vi "UpdateMotors.vi"(0 "I/O":T24 {"IMU SPI A"."SPI Configuration"."Frame Length" min=1 max=16}, 2 "Speed Fraction":dbl min=-1.0 max=1.0 step=0.01, 3 "Spin Fraction":dbl min=-1.0 max=1.0 step=0.001) -> ()   [LabVIEW 2015]
uses:
  <vilib>/myRIO/Instrument Drivers/Onboard IO/PWM/typedefs/PWM Reference.ctl
  <vilib>/myRIO/Common/Instrument Driver Framework/Utilities/typedefs/myRIO Generic Hardware Reference.ctl
  <vilib>/myRIO/Common/Instrument Driver Framework/Utilities/typedefs/Hardware Version Enum.ctl
  <vilib>/myRIO/Common/Instrument Driver Framework/Utilities/typedefs/myRIO v1.0 Reference.ctl
  <vilib>/myRIO/Common/Instrument Driver Framework/Utilities/typedefs/Generic FPGA Reference.ctl
  <vilib>/myRIO/Common/Instrument Driver Framework/myRIO v1.0/PWM/typedefs/PWM Channels Enum.ctl
  <vilib>/myRIO/Instrument Drivers/Onboard IO/PWM/typedefs/PWM Configuration.ctl
  <vilib>/myRIO/Instrument Drivers/Onboard IO/Encoder/typedefs/Encoder Reference.ctl
  <vilib>/myRIO/Common/Instrument Driver Framework/myRIO v1.0/Encoder/typedefs/Encoder Channels Enum.ctl
  <vilib>/myRIO/Instrument Drivers/Onboard IO/SPI/typedefs/SPI Reference.ctl
  <vilib>/myRIO/Common/Instrument Driver Framework/myRIO v1.0/SPI/typedefs/SPI Channels Enum.ctl
  <vilib>/myRIO/Instrument Drivers/Onboard IO/SPI/typedefs/SPI Configuration.ctl
  <vilib>/myRIO/Common/Instrument Driver Framework/myRIO v1.0/SPI/typedefs/SPI Clock Phase.ctl
  <vilib>/myRIO/Common/Instrument Driver Framework/myRIO v1.0/SPI/typedefs/SPI Clock Polarity.ctl
  <vilib>/myRIO/Common/Instrument Driver Framework/myRIO v1.0/SPI/typedefs/SPI Data Direction.ctl
  <vilib>/myRIO/Common/Instrument Driver Framework/myRIO v1.0/SPI/typedefs/SPI Frame Length.ctl
  <vilib>/myRIO/Instrument Drivers/Onboard IO/DIO/typedefs/DIO Reference.ctl
  <vilib>/myRIO/Common/Instrument Driver Framework/myRIO v1.0/DIO/typedefs/DIO Channels List.ctl
  <vilib>/myRIO/Common/Instrument Driver Framework/myRIO v1.0/DIO/typedefs/DIO Channels Enum.ctl
  <vilib>/myRIO/Instrument Drivers/Onboard IO/I2C/typedefs/I2C Reference.ctl
  <vilib>/myRIO/Common/Instrument Driver Framework/myRIO v1.0/I2C/typedefs/I2C Channels Enum.ctl
  <vilib>/myRIO/Instrument Drivers/Onboard IO/I2C/typedefs/I2C Configuration.ctl
  <vilib>/myRIO/Instrument Drivers/Onboard IO/I2C/typedefs/I2C Transfer Rate.ctl
  <vilib>/myRIO/Instrument Drivers/Onboard IO/PWM/vis/Set Duty Cycle and Frequency.vi
  <vilib>/Utility/error.llb/Error Cluster From Error Code.vi
  <vilib>/myRIO/Common/Instrument Driver Framework/myRIO v1.0/PWM/vis/myRIO v1.0 Write PWM.vi
  <vilib>/myRIO/Instrument Drivers/Onboard IO/PWM/PWM.lvlib
  <vilib>/myRIO/Instrument Drivers/Onboard IO/I2C/I2C.lvlib
  <vilib>/myRIO/Instrument Drivers/Onboard IO/DIO/DIO.lvlib
  <vilib>/myRIO/Instrument Drivers/Onboard IO/SPI/SPI.lvlib
  <vilib>/myRIO/Instrument Drivers/Onboard IO/Encoder/Encoder.lvlib
panel:
  out "Array of RMotF and LMotF":dbl[][](array[numeric]) format="%#_2g"
  out "R Mot F":dbl(graph)
  out "L Mot F":dbl(graph)
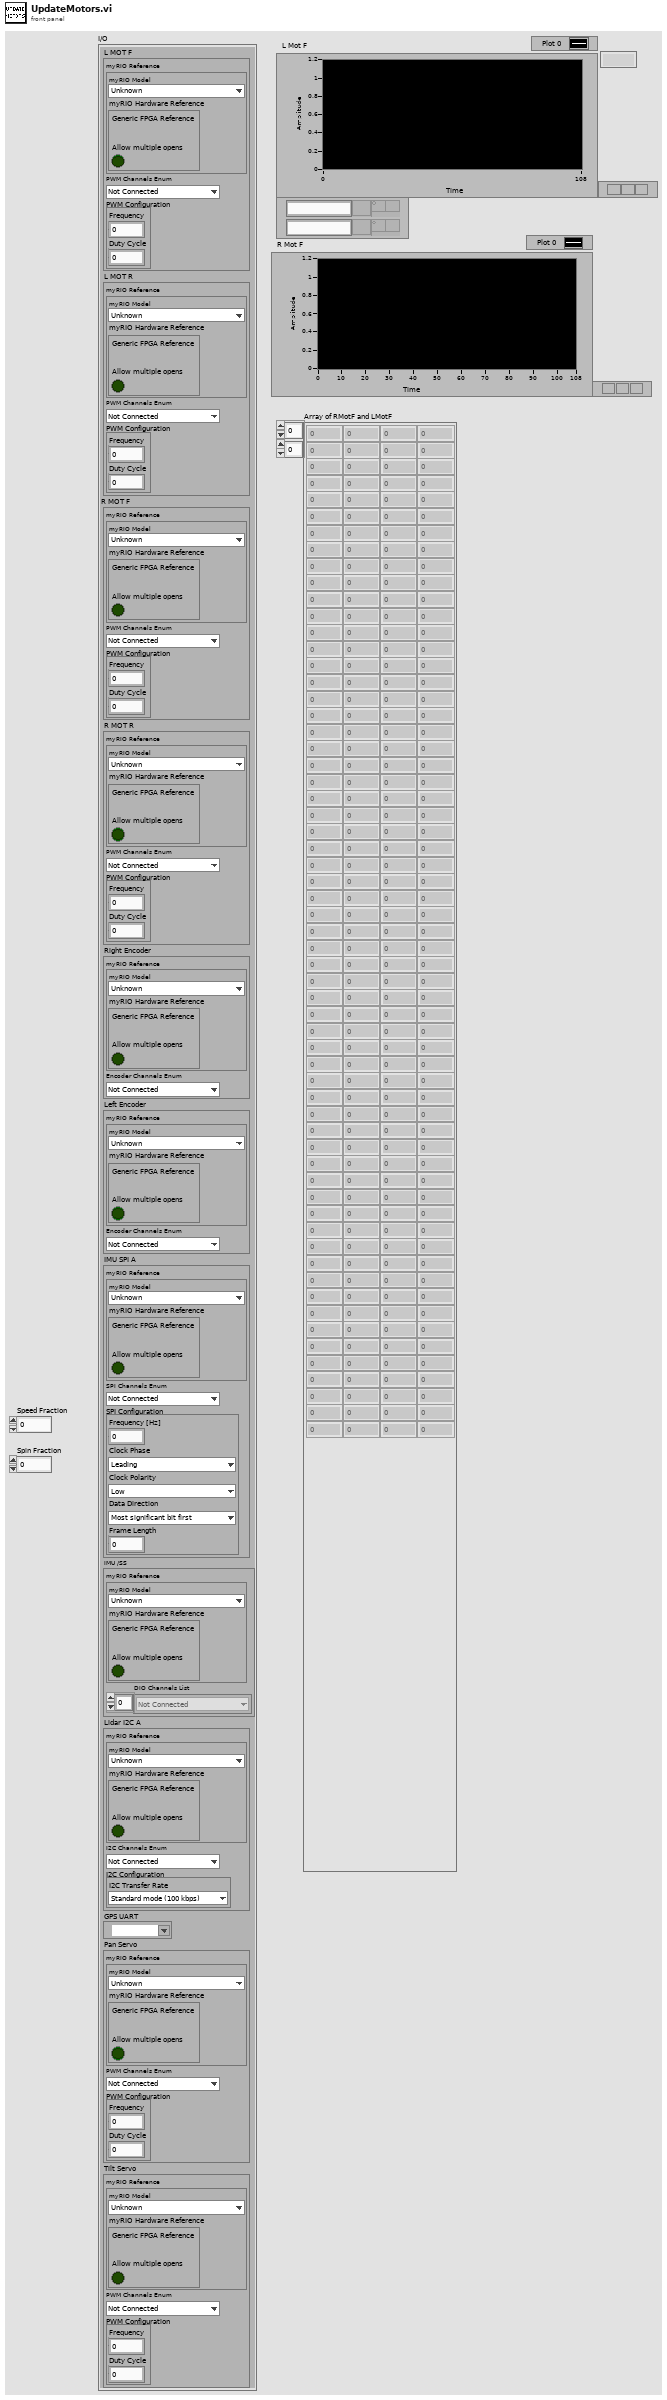
[diagram p1: front panel]
types:
  T1 = typedef "PWM.lvlib/PWM Reference.ctl" = cluster{"myRIO Reference":T2, "PWM Channels Enum":T6, "PWM Configuration":T7}
  T2 = typedef "myRIO Generic Hardware Reference.ctl" = cluster{"myRIO Model":T3, "myRIO Hardware Reference":T4}
  T3 = typedef "Hardware Version Enum.ctl" = enum16{"Unknown", "myRIO-1900", "myRIO-1950", "roboRIO"}
  T4 = typedef "myRIO v1.0 Reference.ctl" = cluster{"Generic FPGA Reference":T5, "Allow multiple opens":bool}
  T5 = typedef "Generic FPGA Reference.ctl" = refnum<k20>
  T6 = typedef "PWM Channels Enum.ctl" = enum16{"Not Connected", "C/PWM0", "C/PWM1", "A/PWM0", "A/PWM1", "A/PWM2", "B/PWM0", "B/PWM1", "B/PWM2", "PWM/PWM0", "PWM/PWM1", "PWM/PWM2", "PWM/PWM3", "PWM/PWM4", "PWM/PWM5", "PWM/PWM6", "PWM/PWM7", "PWM/PWM8", "PWM/PWM9"}
  T7 = typedef "PWM.lvlib/PWM Configuration.ctl" = cluster{"Frequency":dbl, "Duty Cycle":dbl}
  T8 = typedef "Encoder.lvlib/Encoder Reference.ctl" = cluster{"myRIO Reference":T2, "Encoder Channels Enum":T9}
  T9 = typedef "Encoder Channels Enum.ctl" = enum16{"Not Connected", "C/ENC0", "C/ENC1", "A/ENC", "B/ENC", "DIO/ENC0", "DIO/ENC1", "DIO/ENC2", "DIO/ENC3", "DIO/ENC4"}
  T10 = typedef "SPI.lvlib/SPI Reference.ctl" = cluster{"myRIO Reference":T2, "SPI Channels Enum":T11, "SPI Configuration":T12}
  T11 = typedef "SPI Channels Enum.ctl" = enum16{"Not Connected", "A/SPI", "B/SPI", "SPI/SPI"}
  T12 = typedef "SPI.lvlib/SPI Configuration.ctl" = cluster{"Frequency [Hz]":dbl, "Clock Phase":T13, "Clock Polarity":T14, "Data Direction":T15, "Frame Length":T16}
  T13 = typedef "SPI Clock Phase.ctl" = enum8{"Leading", "Trailing"}
  T14 = typedef "SPI Clock Polarity.ctl" = enum8{"Low", "High"}
  T15 = typedef "SPI Data Direction.ctl" = enum8{"Most significant bit first", "Least significant bit first"}
  T16 = typedef "SPI Frame Length.ctl" = u8
  T17 = typedef "DIO.lvlib/DIO Reference.ctl" = cluster{"myRIO Reference":T2, "DIO Channels List":T18}
  T18 = typedef "DIO Channels List.ctl" = T19[]
  T19 = typedef "DIO Channels Enum.ctl" = enum16{"Not Connected", "C/DIO0", "C/DIO1", "C/DIO2", "C/DIO3", "C/DIO4", "C/DIO5", "C/DIO6", "C/DIO7", "A/DIO0", "A/DIO1", "A/DIO2", "A/DIO3", "A/DIO4", "A/DIO5", "A/DIO6", "A/DIO7", "A/DIO8", "A/DIO9", "A/DIO10", "A/DIO11", "A/DIO12", "A/DIO13", "A/DIO14", "A/DIO15", "B/DIO0", "B/DIO1", "B/DIO2", "B/DIO3", "B/DIO4", "B/DIO5", "B/DIO6", "B/DIO7", "B/DIO8", "B/DIO9", "B/DIO10", "B/DIO11", "B/DIO12", "B/DIO13", "B/DIO14", "B/DIO15", "LED0", "LED1", "LED2", "LED3", "Button0", "DIO/DIO0", "DIO/DIO1", "DIO/DIO2", "DIO/DIO3", "DIO/DIO4", "DIO/DIO5", "DIO/DIO6", "DIO/DIO7", "DIO/DIO8", "DIO/DIO9", "SPI/CS0", "SPI/CS1", "SPI/CS2", "SPI/CS3", "LED RADIO (Green)", "LED RADIO (Red)", "LED COMM (Green)", "LED COMM (Red)", "LED MODE (Green)", "LED MODE (Red)"}
  T20 = typedef "I2C.lvlib/I2C Reference.ctl" = cluster{"myRIO Reference":T2, "I2C Channels Enum":T21, "I2C Configuration":T22}
  T21 = typedef "I2C Channels Enum.ctl" = enum16{"Not Connected", "A/I2C", "B/I2C", "I2C/I2C"}
  T22 = typedef "I2C.lvlib/I2C Configuration.ctl" = cluster{"I2C Transfer Rate":T23}
  T23 = typedef "I2C.lvlib/I2C Transfer Rate.ctl" = enum16{"Standard mode (100 kbps)", "Fast mode (400 kbps)"}
  T24 = cluster{"L MOT F":T1, "L MOT R":T1, "R MOT F":T1, "R MOT R":T1, "Right Encoder":T8, "Left Encoder":T8, "IMU SPI A":T10, "IMU /SS":T17, "Lidar I2C A":T20, "GPS UART":refnum<visa-resource-name>, "Pan Servo":T1, "Tilt Servo":T1}
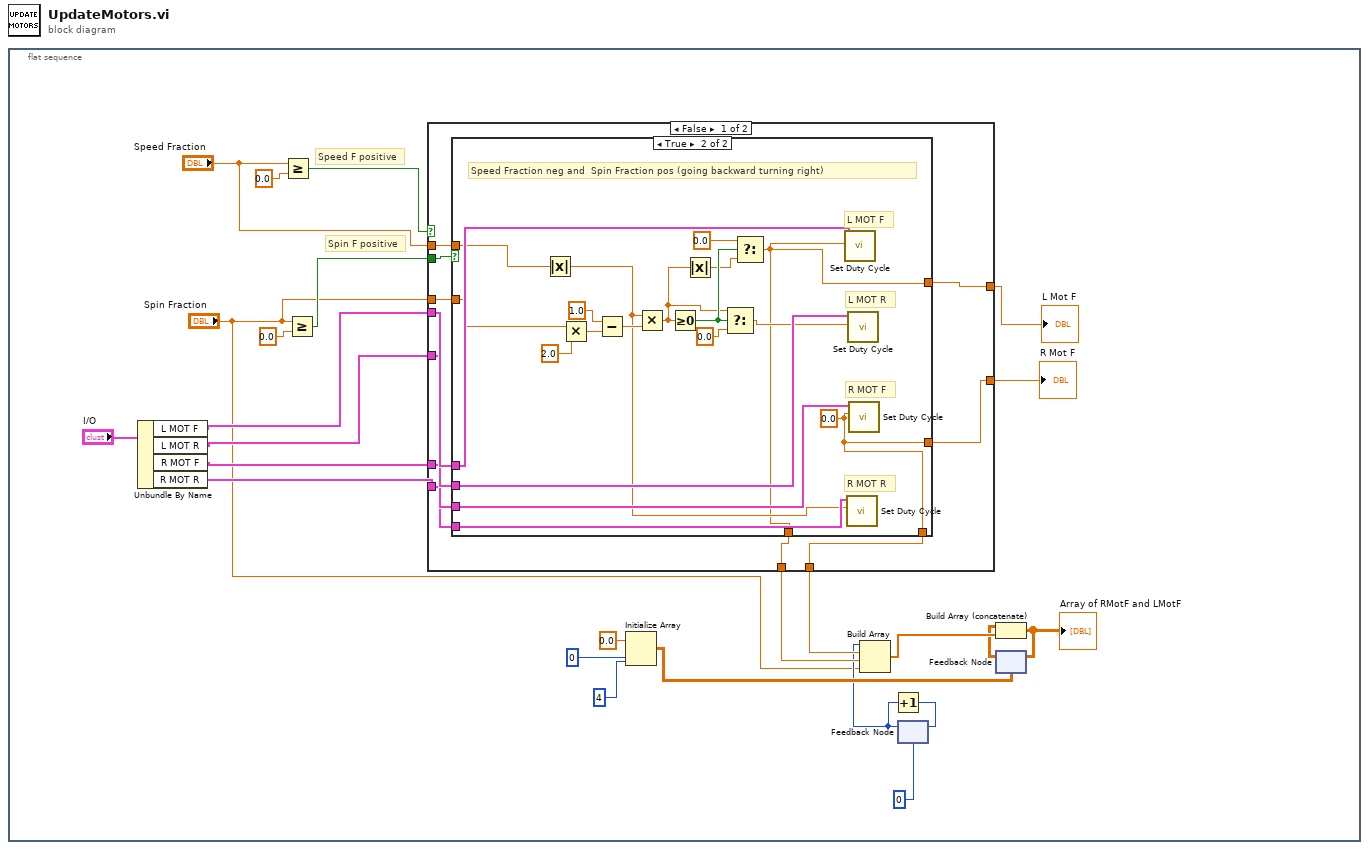
[diagram p0: block diagram]
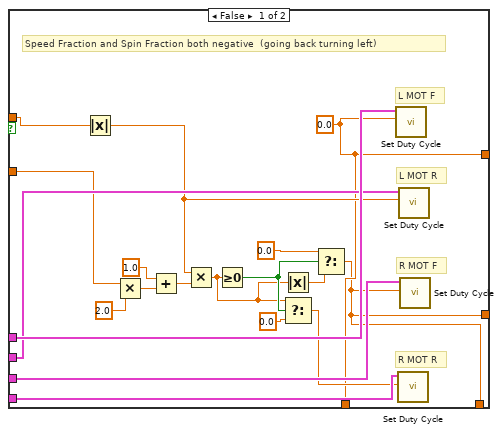
[diagram p2: hidden frame]
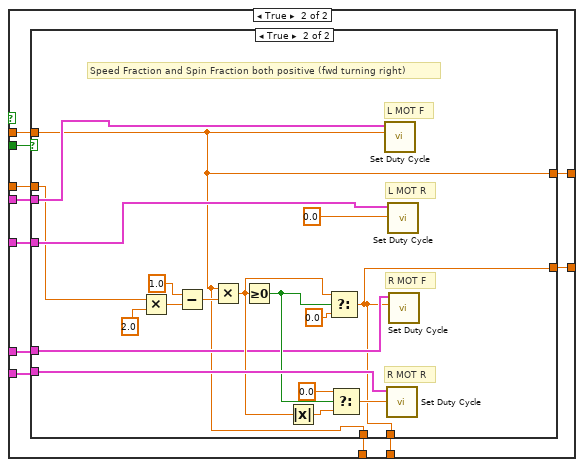
[diagram p3: hidden frame]
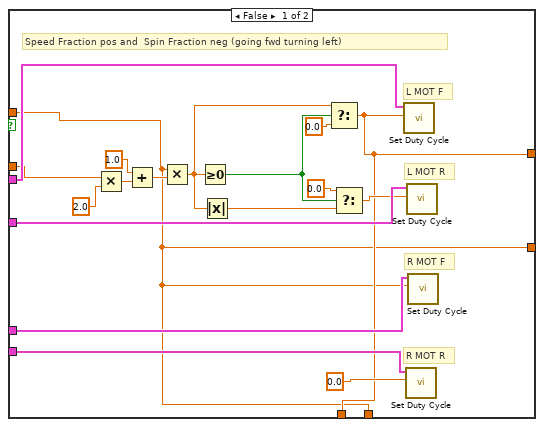
[diagram p4: hidden frame]
diagram:
  n1 = flat-sequence {
    frame #0 {
      # "Spin F positive"
      # "Speed F positive"
      n2 = Unbundle By Name("I/O") -> ("L MOT F"=w20:T1, "L MOT R"=w19:T1, "R MOT F"=w18:T1, "R MOT R"=w17:T1)
      n3 = Greater Or Equal?(x="Speed Fraction", y=0.0) -> (x >= y?=w23:bool)
      n4 = Greater Or Equal?(x="Spin Fraction", y=0.0) -> (x >= y?=w22:bool)
      n5 = case shown="False" w23 {
        tunnel: w22 -> [w36 w85]
        tunnel: w20 -> [w35 w84]
        tunnel: w19 -> [w34 w83]
        tunnel: w18 -> [w33 w82]
        tunnel: w17 -> [w32 w81]
        tunnel: [w31 w80] -> w16
        tunnel: [w30 w79] -> w15
        tunnel: [w28 w78] -> w13
        tunnel: [w29 w77] -> w12
        tunnel: "Speed Fraction" -> [w27 w76]
        tunnel: "Spin Fraction" -> [w26 w75]
        frame False {
          n6 = case shown="True" w36 {
            tunnel: w35 -> [w51 w70]
            tunnel: w34 -> [w50 w69]
            tunnel: w33 -> [w49 w68]
            tunnel: w32 -> [w48 w67]
            tunnel: [w40 w59] -> w31
            tunnel: [w39 w58] -> w30
            tunnel: [w40 w59] -> w29
            tunnel: [w39 w58] -> w28
            tunnel: w27 -> [w38 w57]
            tunnel: w26 -> [w37 w56]
            frame False {
              w40 = 0.0 ("Duty Cycle")
              # "Speed Fraction and Spin Fraction both negative  (going back turning left)"
              # "R MOT R"
              # "L MOT R"
              # "R MOT F"
              # "L MOT F"
              n7 = Absolute Value(x=w38) -> (abs(x)=w47:dbl)
              n8 = Multiply(x=w37, y=2.0) -> (x*y=w53:dbl)
              n9 = Add(x=1.0, y=w53) -> (x+y=w55:dbl)
              n10 = Multiply(x=w47, y=w55) -> (x*y=w42:dbl)
              n11 = Greater Or Equal To 0?(x=w42) -> (x >= 0?=w44:bool)
              n12 = Absolute Value(x=w42) -> (abs(x)=w41:dbl)
              n13 = Select(t=w42, s=w44, f=0.0) -> (s? t:f=w45:dbl)
              n14 = Select(t=0.0 ("Duty Cycle"), s=w44, f=w41) -> (s? t:f=w39:dbl)
              n15 = call <vilib>:"Set Duty Cycle.vi"("Duty Cycle"=w40, "PWM Ref In"=w51) -> ()  [unwired: 7 in, 2 out]
              n16 = call <vilib>:"Set Duty Cycle.vi"("Duty Cycle"=w45, "PWM Ref In"=w48) -> ()  [unwired: 7 in, 2 out]
              n17 = call <vilib>:"Set Duty Cycle.vi"("Duty Cycle"=w47, "PWM Ref In"=w50) -> ()  [unwired: 7 in, 2 out]
              n18 = call <vilib>:"Set Duty Cycle.vi"("Duty Cycle"=w39, "PWM Ref In"=w49) -> ()  [unwired: 7 in, 2 out]
            }
            frame True {
              w58 = 0.0 ("Duty Cycle")
              # "Speed Fraction neg and  Spin Fraction pos (going backward turning right)"
              # "R MOT R"
              # "L MOT R"
              # "R MOT F"
              # "L MOT F"
              n19 = Absolute Value(x=w57) -> (abs(x)=w66:dbl)
              n20 = Multiply(x=w56, y=2.0) -> (x*y=w73:dbl)
              n21 = Subtract(x=1.0, y=w73) -> (x-y=w71:dbl)
              n22 = Multiply(x=w66, y=w71) -> (x*y=w60:dbl)
              n23 = Greater Or Equal To 0?(x=w60) -> (x >= 0?=w62:bool)
              n24 = Absolute Value(x=w60) -> (abs(x)=w61:dbl)
              n25 = Select(t=w60, s=w62, f=0.0) -> (s? t:f=w65:dbl)
              n26 = Select(t=0.0 ("Duty Cycle"), s=w62, f=w61) -> (s? t:f=w59:dbl)
              n27 = call <vilib>:"Set Duty Cycle.vi"("Duty Cycle"=w59, "PWM Ref In"=w70) -> ()  [unwired: 7 in, 2 out]
              n28 = call <vilib>:"Set Duty Cycle.vi"("Duty Cycle"=w66, "PWM Ref In"=w67) -> ()  [unwired: 7 in, 2 out]
              n29 = call <vilib>:"Set Duty Cycle.vi"("Duty Cycle"=w65, "PWM Ref In"=w69) -> ()  [unwired: 7 in, 2 out]
              n30 = call <vilib>:"Set Duty Cycle.vi"("Duty Cycle"=w58, "PWM Ref In"=w68) -> ()  [unwired: 7 in, 2 out]
            }
          }
        }
        frame True {
          n31 = case shown="True" w85 {
            tunnel: w84 -> [w98 w116]
            tunnel: w83 -> [w97 w115]
            tunnel: w82 -> [w96 w107]
            tunnel: w81 -> [w95 w114]
            tunnel: [w88 w104] -> w80
            tunnel: [w87 w106] -> w79
            tunnel: [w87 w106] -> w78
            tunnel: [w88 w104] -> w77
            tunnel: w76 -> [w87 w104]
            tunnel: w75 -> [w86 w105]
            frame False {
              # "Speed Fraction pos and  Spin Fraction neg (going fwd turning left)"
              # "R MOT R"
              # "L MOT R"
              # "R MOT F"
              # "L MOT F"
              n32 = Multiply(x=w86, y=2.0) -> (x*y=w102:dbl)
              n33 = Add(x=1.0, y=w102) -> (x+y=w100:dbl)
              n34 = Multiply(x=w87, y=w100) -> (x*y=w90:dbl)
              n35 = Greater Or Equal To 0?(x=w90) -> (x >= 0?=w92:bool)
              n36 = Absolute Value(x=w90) -> (abs(x)=w89:dbl)
              n37 = Select(t=w90, s=w92, f=0.0) -> (s? t:f=w88:dbl)
              n38 = Select(t=0.0, s=w92, f=w89) -> (s? t:f=w93:dbl)
              n39 = call <vilib>:"Set Duty Cycle.vi"("Duty Cycle"=w88, "PWM Ref In"=w98) -> ()  [unwired: 7 in, 2 out]
              n40 = call <vilib>:"Set Duty Cycle.vi"("Duty Cycle"=0.0, "PWM Ref In"=w95) -> ()  [unwired: 7 in, 2 out]
              n41 = call <vilib>:"Set Duty Cycle.vi"("Duty Cycle"=w93, "PWM Ref In"=w97) -> ()  [unwired: 7 in, 2 out]
              n42 = call <vilib>:"Set Duty Cycle.vi"("Duty Cycle"=w87, "PWM Ref In"=w96) -> ()  [unwired: 7 in, 2 out]
            }
            frame True {
              # "Speed Fraction and Spin Fraction both positive (fwd turning right)"
              # "R MOT R"
              # "L MOT R"
              # "R MOT F"
              # "L MOT F"
              n43 = Multiply(x=w105, y=2.0) -> (x*y=w120:dbl)
              n44 = Subtract(x=1.0, y=w120) -> (x-y=w118:dbl)
              n45 = Multiply(x=w104, y=w118) -> (x*y=w109:dbl)
              n46 = Greater Or Equal To 0?(x=w109) -> (x >= 0?=w112:bool)
              n47 = Absolute Value(x=w109) -> (abs(x)=w110:dbl)
              n48 = Select(t=w109, s=w112, f=0.0) -> (s? t:f=w106:dbl)
              n49 = Select(t=0.0, s=w112, f=w110) -> (s? t:f=w108:dbl)
              n50 = call <vilib>:"Set Duty Cycle.vi"("Duty Cycle"=w104, "PWM Ref In"=w116) -> ()  [unwired: 7 in, 2 out]
              n51 = call <vilib>:"Set Duty Cycle.vi"("Duty Cycle"=w108, "PWM Ref In"=w114) -> ()  [unwired: 7 in, 2 out]
              n52 = call <vilib>:"Set Duty Cycle.vi"("Duty Cycle"=0.0, "PWM Ref In"=w115) -> ()  [unwired: 7 in, 2 out]
              n53 = call <vilib>:"Set Duty Cycle.vi"("Duty Cycle"=w106, "PWM Ref In"=w107) -> ()  [unwired: 7 in, 2 out]
            }
          }
        }
      }
      "L Mot F" <- w16
      "R Mot F" <- w15
      n54 = Initialize Array(0.0 ("element"), 0 ("dimension size"), 4 ("dimension size")) -> (w7:dbl[][])
      n55 = feedback #1(0) -> (w3:i32)
      n56 = Build Array(w3, w13, w12, "Spin Fraction") -> (w14:dbl[])
      n57 = Increment(x=w3) -> (x+1=w4:i32)
      n58 = feedback-in #1(w4) -> ()
      n59 = feedback #2(w7) -> (w11:dbl[][])
      n60 = Build Array (concatenate)(w11, w14) -> (w6:dbl[][])
      "Array of RMotF and LMotF" <- w6
      n61 = feedback-in #2(w6) -> ()
    }
  }
